vi "Embedded TDMS Logger.Async.vi"(10 "Parameters":variant, 11 "Process":refnum<class "Process.lvclass">) -> ()   [LabVIEW 2024, in "Embedded TDMS Logger Engine.lvlib"]
doc: "The Asynchronous VI for our Custom Device, it is the main loop and uses the Channel Manager class to handle most of the logic. This is the Engine for our Embedded TDMS Logger and handles the following tasks:\n- Setup and get the Wfm Sessions\n- Read our Channel data from the RT Driver\n- Are we triggered?:\n - Do we need to open a new file, close the current file or do nothing?\n- Log the data or not\n- Check whether to segment the file and if so, close the current file and reopen.\n- Log data back to the user channels.\n- Close the file cleanly"
uses:
  Embedded TDMS Logger Engine.lvlib
  <vilib>/NI/NIVS Inline Async API/_VS Inline Async API/Process/Process.lvclass
  Shared/Compiled.Settings.ctl
  Shared/SegmentOptions.ctl
  Shared/File Classes/File/FileAsCluster.ctl
  Shared/File Classes/Group/GroupAsCluster.ctl
  Shared/File Classes/Channel/ChannelAsCluster.ctl
  <vilib>/NI VeriStand/Custom Device API/Data Reference.ctl
  Shared/File Classes/Meta Data.ctl
  <vilib>/NI/NIVS Inline Async API/_VS Inline Async API/Process/Process.lvclass/Process.ctl
  <vilib>/NI/NIVS Inline Async API/_VS Inline Async API/Process/Data Member Access/Read Data Access.vi
  <vilib>/NI/NIVS Inline Async API/_VS Inline Async API/Error Handling Process/SubVIs/Error.ConvertArray.vi
  <vilib>/NI/NIVS Inline Async API/_Data Access Engine/Data Access Engine/Data Access Engine.lvclass
  Channel Reader/Channel Manager.lvclass
  Shared/Embedded TDMS Logger Shared.lvlib
  <vilib>/NI VeriStand/Custom Device API/Custom Device API.lvlib
panel:
  out "data":T1={"Name"="", "Async Init Timeout"=0, "Segment Files"=FALSE, "Segment Every"=0.0, "Segment by"=enum."Size (MB)", "dt per loop"=0.0, "output cluster"={"Name"="", "Directory"="", "Date Captured"="", "Groups"=[], "Meta Data"=[], "File Start Time"=timestamp(0 s since 1904-01-01), "appended path"=path ""}} {"output cluster"."Groups"."Channels"."Data Reference" format="%.0x"}
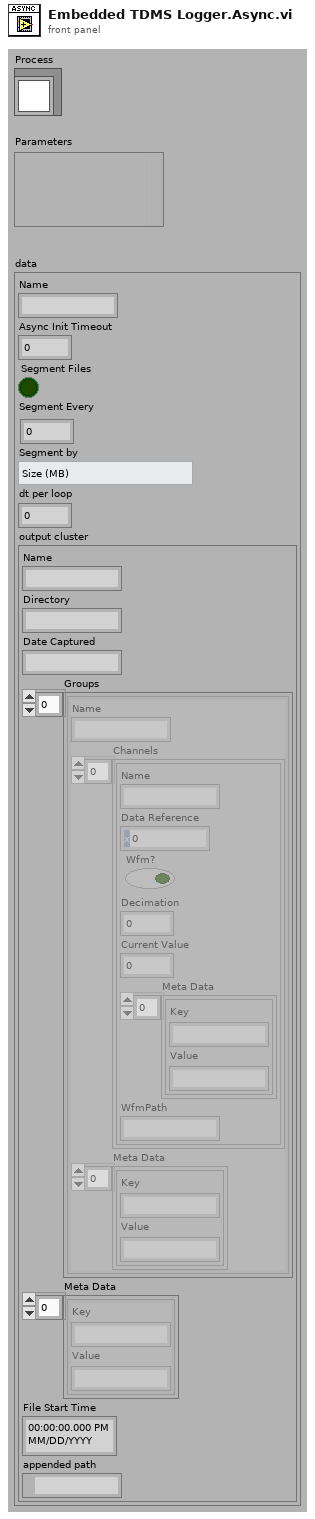
[diagram p1: front panel]
types:
  T1 = typedef "Embedded TDMS Logger Shared.lvlib/Compiled.Settings.ctl" = cluster{"Name":string, "Async Init Timeout":u16, "Segment Files":bool, "Segment Every":dbl, "Segment by":T2, "dt per loop":dbl, "output cluster":T3}
  T2 = typedef "SegmentOptions.ctl" = enum16{"Time (s)", "Size (MB)"}
  T3 = typedef "FileAsCluster.ctl" = cluster{"Name":string, "Directory":string, "Date Captured":string, "Groups":T4[], "Meta Data":T7[], "File Start Time":timestamp, "appended path":path}
  T4 = typedef "GroupAsCluster.ctl" = cluster{"Name":string, "Channels":T5[], "Meta Data":T7[]}
  T5 = typedef "ChannelAsCluster.ctl" = cluster{"Name":string, "Data Reference":T6, "Wfm?":bool, "Decimation":i32, "Current Value":dbl, "Meta Data":T7[], "WfmPath":string}
  T6 = typedef "Custom Device API.lvlib/Data Reference.ctl" = i32
  T7 = typedef "Meta Data.ctl" = cluster{"Key":string, "Value":string}
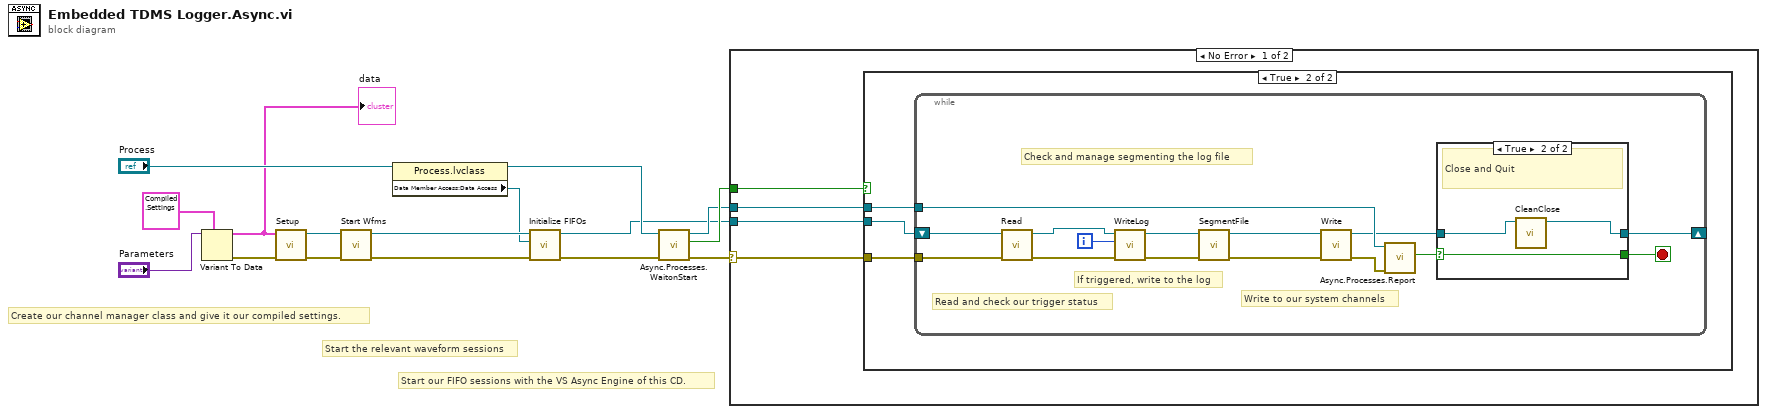
[diagram p0: block diagram]
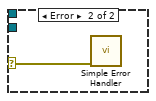
[diagram p4: hidden frame]
diagram:
  # "Start our FIFO sessions with the VS Async Engine of this CD."
  # "Start the relevant waveform sessions"
  # "Create our channel manager class and give it our compiled settings."
  n1 = Variant To Data(type=T1 {"Name"="", "Async Init Timeout"=0, "Segment Files"=FALSE, "Segment Every"=0.0, "Segment by"=enum."Size (MB)", "dt per loop"=0.0, "output cluster"={"Name"="", "Directory"="", "Date Captured"="", "Groups"=[], "Meta Data"=[], "File Start Time"=timestamp(0 s since 1904-01-01), "appended path"=path ""}} ("Compiled.Settings"), Variant="Parameters") -> (data=w7:T1, error out=w2:errorcluster)  [unwired: 1 in]
  "data" <- w7
  n2 = call "Setup.vi"("error in (no error)"=w2, "Compiled Data In"=w7) -> ("error out"=w1:errorcluster, "Channel Manager out"=w10:refnum<class "Channel Manager.lvclass">)  [unwired: 8 in]
  n3 = call-dynamic "Start Wfms.vi"("error in (no error)"=w1, "Channel Manager in"=w10) -> ("error out"=w8:errorcluster, "Channel Manager out"=w9:refnum<class "Channel Manager.lvclass">)  [unwired: 8 in]
  n4 = property class="Process.lvclass"(reference="Process") -> (reference out=w13:refnum<class "Process.lvclass">, "Data Member Access:Data Access"=w6:refnum<class "Data Access Engine.lvclass">)  [unwired: 1 in, 1 out]
  n5 = call-dynamic "Initialize FIFOs.vi"("error in (no error)"=w8, "Data Access"=w6, "Channel Reader in"=w9) -> ("error out"=w3:errorcluster, "Channel Reader out"=w4:refnum<class "Channel Manager.lvclass">)  [unwired: 7 in]
  n6 = call <vilib>:"Async.Processes.WaitonStart.vi"("error in (no error)"=w3, "Process"=w13) -> ("error out"=w5:errorcluster, "Execute"=w16:bool, "Process out"=w15:refnum<class "Process.lvclass">)  [unwired: 7 in]
  n7 = case shown="No Error" w5 {
    selector: w5 -> [w18 w44]
    tunnel: w16 -> [w20 _]
    tunnel: w15 -> [w19 _]
    tunnel: w4 -> [w17 _]
    frame No Error {
      n8 = case shown="True" w20 {
        tunnel: w18 -> [_ w22]
        tunnel: w19 -> [_ w23]
        tunnel: w17 -> [_ w21]
        frame False {
        }
        frame True {
          n9 = while {
            tunnel: w22 -> [w25]
            tunnel: w23 -> [w38]
            shift-right: [w32] -> _
            shift-left: w21 -> [w31]
            i -> [w35]
            stop <- w36 stop-if-true
            # "Write to our system channels"
            # "Check and manage segmenting the log file"
            # "If triggered, write to the log"
            # "Read and check our trigger status"
            n10 = call-dynamic "Read.vi"("error in (no error)"=w25, "Channel Reader in"=w31) -> ("error out"=w26:errorcluster, "Channel Reader out"=w30:refnum<class "Channel Manager.lvclass">)  [unwired: 8 in]
            n11 = call-dynamic "WriteLog.vi"("error in (no error)"=w26, "Loop Counter"=w35, "Channel Manager in"=w30) -> ("error out"=w27:errorcluster, "Channel Manager out"=w29:refnum<class "Channel Manager.lvclass">)  [unwired: 7 in]
            n12 = call-dynamic "SegmentFile.vi"("error in (no error)"=w27, "Channel Manager in"=w29) -> ("error out"=w28:errorcluster, "Channel Manager out"=w34:refnum<class "Channel Manager.lvclass">)  [unwired: 8 in]
            n13 = call-dynamic "Write.vi"("error in (no error)"=w28, "Channel Manager in"=w34) -> ("error out"=w24:errorcluster, "Channel Manager out"=w33:refnum<class "Channel Manager.lvclass">)  [unwired: 8 in]
            n14 = call <vilib>:"Async.Processes.Report.vi"("Error"=w24, "Process in"=w38) -> ("Stop"=w37:bool)  [unwired: 8 in, 1 out]
            n15 = case shown="True" w37 {
              selector: w37 -> [w40 w43]
              tunnel: [w40 w43] -> w36
              tunnel: w33 -> [w39 w42]
              tunnel: [w39 w41] -> w32
              frame False {
              }
              frame True {
                # "Close and Quit"
                n16 = call-dynamic "CleanClose.vi"("Channel Manager in"=w42) -> ("Channel Manager out"=w41:refnum<class "Channel Manager.lvclass">)  [unwired: 9 in, 1 out]
              }
            }
          }
        }
      }
    }
    frame Error {
      n17 = call <vilib>:"Simple Error Handler.vi"("error in (no error)"=w44) -> ()  [unwired: 4 in, 5 out]
    }
  }
